vi "10进制转26进制.vi"(1 "十进制":i32) -> (0 "26进制":string)   [LabVIEW 2021, in "OperateExcel.lvlib"]
uses:
  OperateExcel.lvlib
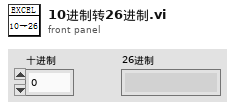
[diagram p1: front panel]
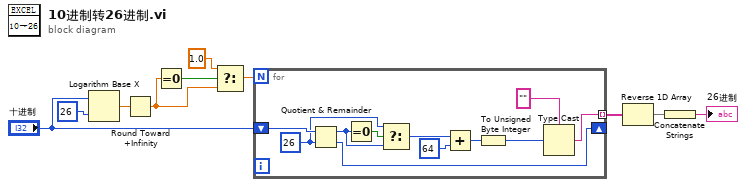
[diagram p0: block diagram]
diagram:
  n1 = Logarithm Base X(1:26 ("x"), 2:"十进制") -> (0:w5:dbl)
  n2 = Round Toward +Infinity(x=w5) -> (ceil(x): smallest int >= x=w3:dbl)
  n3 = Equal To 0?(x=w3) -> (x = 0?=w4:bool)
  n4 = Select(t=1.0, s=w4, f=w3) -> (s? t:f=w1:dbl)
  n5 = for {
    N: w1 -> [_]
    tunnel: [w19] -> w10 mode=indexing
    shift-right: [w16] -> _
    shift-left: "十进制" -> [w21]
    w12 = 26 ("y")
    n6 = Quotient & Remainder(x=w21, y=w12) -> (x-y*floor(x/y)=w13:i32, floor(x/y)=w16:i32)
    n7 = Equal To 0?(x=w13) -> (x = 0?=w14:bool)
    n8 = Select(t=w12, s=w14, f=w13) -> (s? t:f=w11:i32)
    n9 = Add(x=w11, y=64) -> (x+y=w18:i32)
    n10 = To Unsigned Byte Integer(number=w18) -> (unsigned 8bit integer=w17:u8)
    n11 = Type Cast(type="" ("类型"), x=w17) -> (*(type *) &x=w19:string)
  }
  n12 = Reverse 1D Array(array=w10) -> (reversed array=w9:string[])
  n13 = Concatenate Strings(w9) -> (→"26进制":string)
